vi "GT Set Laser Follow Spline.vi"(0 "cardNum":i16, 1 "pY":dbl, 2 "endValue":dbl, 5 "tableId":i16, 7 "n":i32, 9 "pX":dbl, 11 "error in (no error)":errorcluster caption="错误输入（无错误）", 12 "beginValue":dbl, 13 "channel":i16) -> (3 "pY out":dbl, 4 "function return":i16, 10 "pX out":dbl, 15 "error out":errorcluster caption="错误输出")   [LabVIEW 2014, in "gts.lvlib"]
doc: "GT_API GT_SetLaserFollowSpline(short cardNum,short tableId,long n,double *pX,double *pY,double beginValue,double endValue,short channel=0);"
uses:
  gts.lvlib
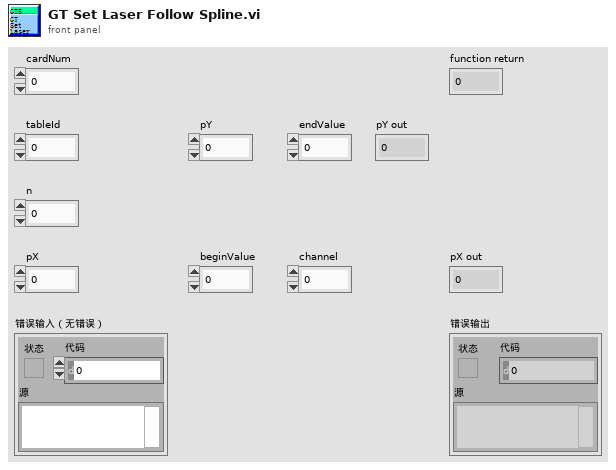
[diagram p1: front panel]
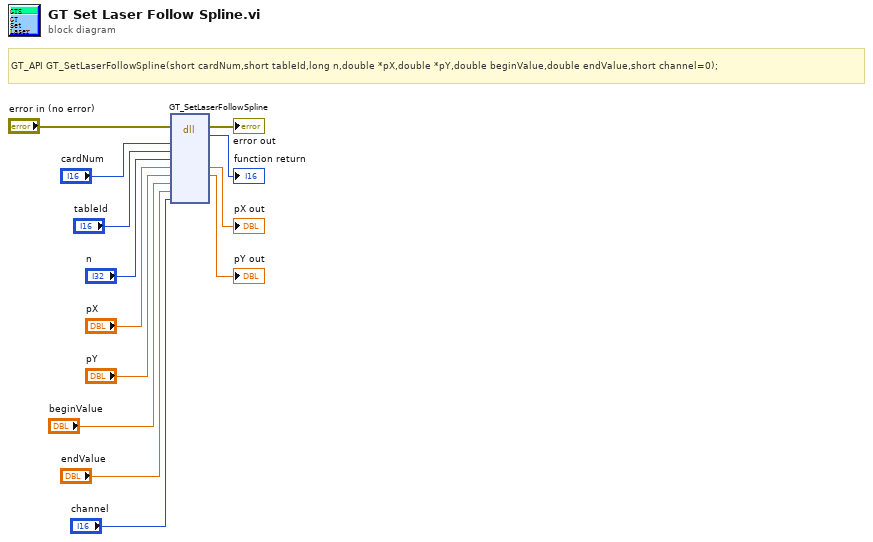
[diagram p0: block diagram]
diagram:
  # "GT_API GT_SetLaserFollowSpline(short cardNum,short tableId,long n,double *pX,double *pY,double beginValue,double endValue,short channel=0);"
  n1 = dll-call lib="PTH2habs D固高科技资料GTS控制卡GTS卡18年上半年资料dllVC32bit\nmulti_cardgts.*" fn="GT_SetLaserFollowSpline"(error in="error in (no error)", "cardNum"="cardNum", "tableId"="tableId", "n"="n", "pX"="pX", "pY"="pY", "beginValue"="beginValue", "endValue"="endValue", "channel"="channel") -> (error out=→"error out":errorcluster, →"function return":i16, "pX"=→"pX out":dbl, "pY"=→"pY out":dbl)  [unwired: 8 in, 1 out]
